vi "右启动扫码全局.vi"() -> ()   [LabVIEW 2014]
panel:
  in  "右启动扫码全局":bool
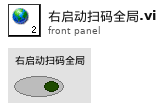
[diagram p1: front panel]
diagram:
